vi "Set-application-path.vi"(8 "error in (no error)":errorcluster, 10 "Main VI ref":refnum<vi>, 11 "Data ref. in":T1) -> (0 "error out":errorcluster, 3 "Data ref.":T1)   [LabVIEW 2013, in "SLMControl.lvlib" / "SC-Main.lvclass"]
uses:
  SC-Main.lvclass
  Object-reference.ctl
  SC-Main.lvclass/SC-Main.ctl
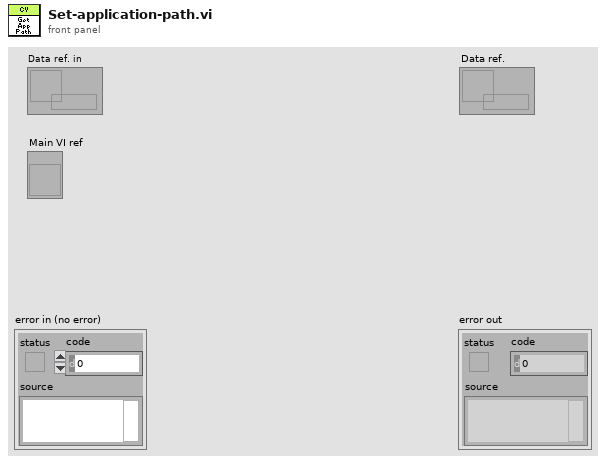
[diagram p1: front panel]
types:
  T1 = typedef "SLMControl.lvlib/SC-Main.lvclass/Object-reference.ctl" = refnum<data-value>
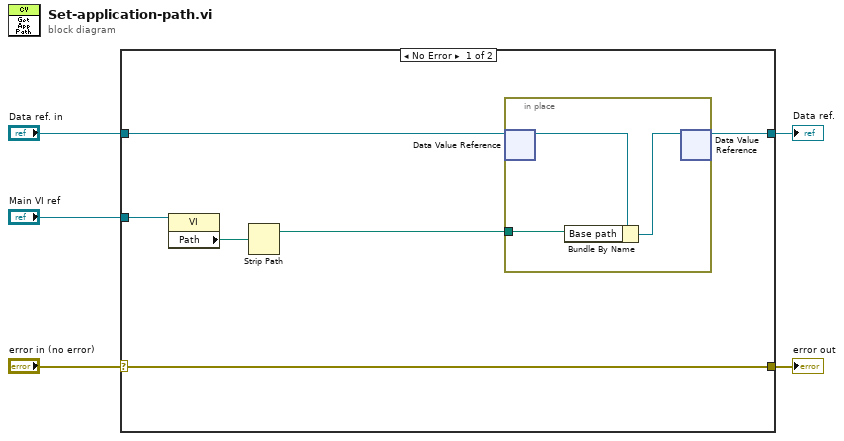
[diagram p0: block diagram]
diagram:
  n1 = case shown="No Error" "error in (no error)" {
    selector: "error in (no error)" -> [w11 w16]
    tunnel: [w11 w16] -> w4
    tunnel: "Data ref. in" -> [w7 w15]
    tunnel: [w8 w15] -> w2
    tunnel: "Main VI ref" -> [w10 _]
    frame No Error {
      n2 = property class="VI"(reference=w10) -> ("Path"=w9:path)  [unwired: 1 in, 2 out]
      n3 = Strip Path(path=w9) -> (stripped path=w6:path)  [unwired: 1 out]
      n4 = in-place {
        in-place-border: w6 -> [w14]
        n5 = in-place-dvr #1(w7) -> (w12:refnum<class "SC-Main.lvclass">)  [unwired: 1 out]
        n6 = Bundle By Name(cluster=w12, "Base path"=w14) -> (w13:refnum<class "SC-Main.lvclass">)
        n7 = in-place-dvr #1(w13) -> (w8:T1)  [unwired: 1 out]
      }
    }
    frame Error {
    }
  }
  "error out" <- w4
  "Data ref." <- w2
